vi "find_close_point_on_line.vi"(9 "Array in":dbl[][](array[numeric]), 10 "fitting axis":dbl, 11 "fitting array":dbl[][](array[numeric])) -> (0 "d":ext, 2 "XY online":dbl[](array[numeric]), 3 "XY point":dbl[](array[numeric]))   [LabVIEW 2017]
uses:
  <vilib>/Analysis/NI_AALPro.lvlib
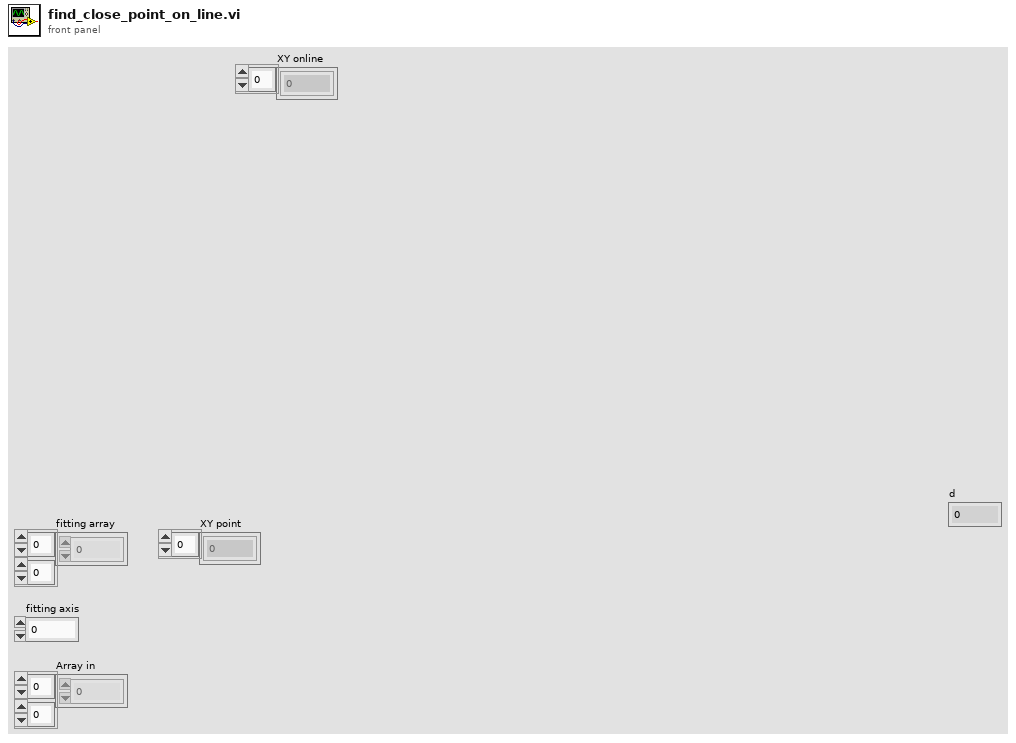
[diagram p1: front panel]
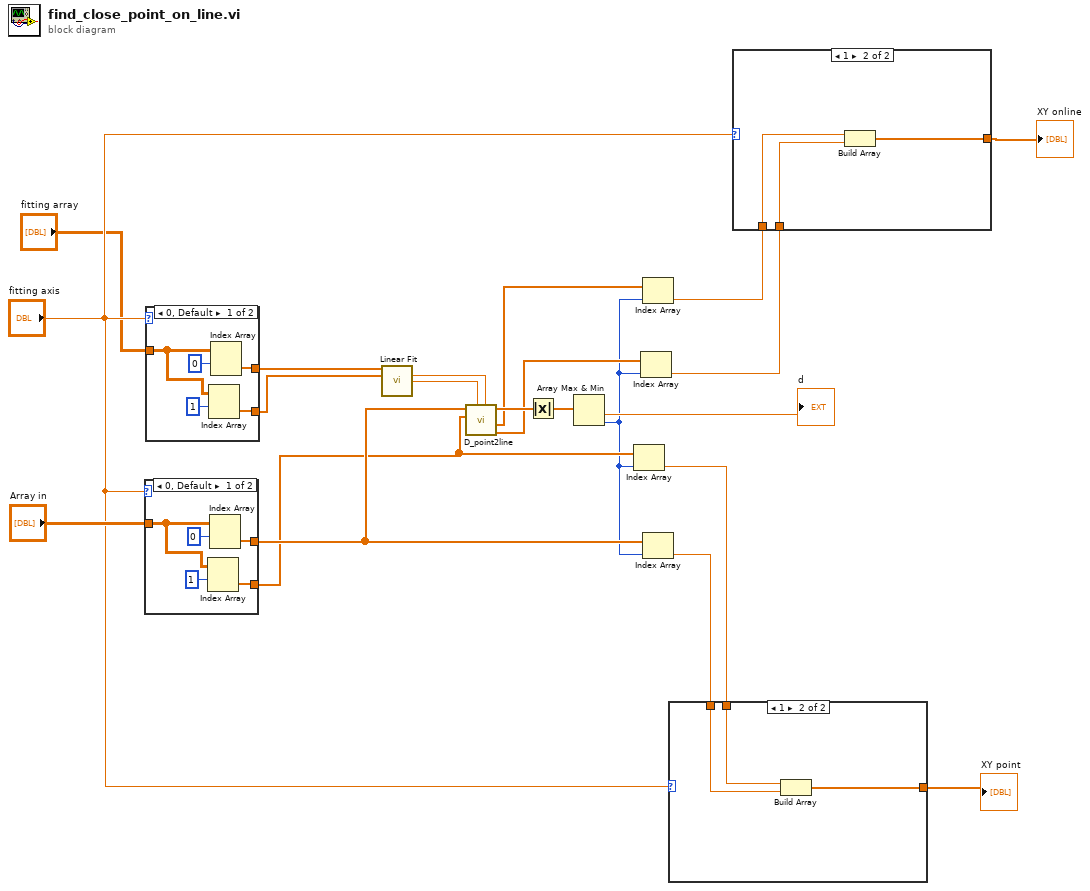
[diagram p0: block diagram]
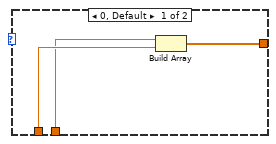
[diagram p2: hidden frame]
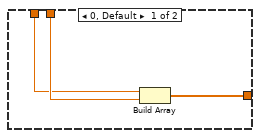
[diagram p3: hidden frame]
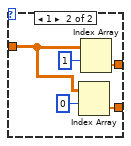
[diagram p4: hidden frame]
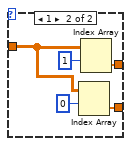
[diagram p5: hidden frame]
diagram:
  n1 = case shown="0, Default" "fitting axis" {
    tunnel: "Array in" -> [w24 w29]
    tunnel: [w23 w28] -> w13
    tunnel: [w22 w27] -> w12
    frame 0, Default {
      n2 = Index Array(array=w24, index (row)=1) -> (element=w22:dbl[])  [unwired: 1 in]
      n3 = Index Array(array=w24, index (row)=0) -> (element=w23:dbl[])  [unwired: 1 in]
    }
    frame 1 {
      n4 = Index Array(array=w29, index (row)=0) -> (element=w27:dbl[])  [unwired: 1 in]
      n5 = Index Array(array=w29, index (row)=1) -> (element=w28:dbl[])  [unwired: 1 in]
    }
  }
  n6 = case shown="0, Default" "fitting axis" {
    tunnel: "fitting array" -> [w34 w39]
    tunnel: [w33 w38] -> w10
    tunnel: [w32 w37] -> w9
    frame 0, Default {
      n7 = Index Array(array=w34, index (row)=1) -> (element=w32:dbl[])  [unwired: 1 in]
      n8 = Index Array(array=w34, index (row)=0) -> (element=w33:dbl[])  [unwired: 1 in]
    }
    frame 1 {
      n9 = Index Array(array=w39, index (row)=0) -> (element=w37:dbl[])  [unwired: 1 in]
      n10 = Index Array(array=w39, index (row)=1) -> (element=w38:dbl[])  [unwired: 1 in]
    }
  }
  n11 = call <vilib>:"Linear Fit.vi"("Y"=w10, "X"=w9) -> ("slope"=w16:dbl, "intercept"=w15:dbl)  [unwired: 9 in, 3 out]
  n12 = call "D_point2line.vi"("slope"=w16, "intercept"=w15, "X Array"=w12, "Y Array"=w13) -> ("Y_online"=w7:ext[], "X_online"=w8:ext[], "D"=w17:ext[])  [unwired: 5 in]
  n13 = Absolute Value(x=w17) -> (abs(x)=w18:ext[])
  n14 = Array Max & Min(array=w18) -> (min value=→"d":ext, min index (indices)=w6:i32)  [unwired: 2 out]
  n15 = Index Array "Index Array"(array=w12, index=w6) -> (element=w19:dbl)
  n16 = Index Array "Index Array"(array=w7, index=w6) -> (element=w3:ext)
  n17 = Index Array "Index Array"(array=w8, index=w6) -> (element=w4:ext)
  n18 = Index Array "Index Array"(array=w13, index=w6) -> (element=w20:dbl)
  n19 = case shown="1" "fitting axis" {
    tunnel: [w44 w47] -> w21
    tunnel: w20 -> [w42 w46]
    tunnel: w19 -> [w43 w45]
    frame 0, Default {
      n20 = Build Array(w42, w43) -> (w44:dbl[])
    }
    frame 1 {
      n21 = Build Array(w45, w46) -> (w47:dbl[])
    }
  }
  "XY point" <- w21
  n22 = case shown="1" "fitting axis" {
    tunnel: [w50 w53] -> w5
    tunnel: w3 -> [w48 w52]
    tunnel: w4 -> [w49 w51]
    frame 0, Default {
      n23 = Build Array(w48, w49) -> (w50:ext[])
    }
    frame 1 {
      n24 = Build Array(w51, w52) -> (w53:ext[])
    }
  }
  "XY online" <- w5
